vi "Start Trial Assert.vi"(8 "error in":errorcluster, 11 "FPGA VI Ref":T1) -> (0 "error out":errorcluster, 3 "FPGA VI Reference Out":T1)   [LabVIEW 2020]
uses:
  RIG-SPECIFIC FILES/FPGA Refs/FPGA Ref.ctl
  <vilib>/Utility/error.llb/Error Cluster From Error Code.vi
  <vilib>/rvi/errors/niLvFpgaAdjustHostInterfaceError.vi
  <vilib>/rvi/interface/nirviReadWriteControl/nirviReadWriteControl.xnode
  <vilib>/rvi/interface/Simulation/niFpgaSimulationCallBeginRW.vi
  NiFpgaLv.dll
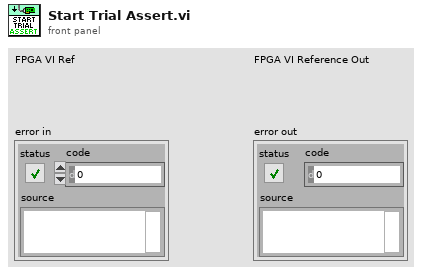
[diagram p1: front panel]
types:
  T1 = typedef "FPGA Ref.ctl" = refnum<k20>
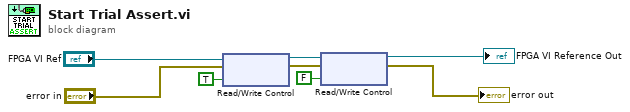
[diagram p0: block diagram]
diagram:
  n1 = xnode "Read/Write Control"("FPGA VI Reference In"="FPGA VI Ref", "error in"="error in", "start_trial"=TRUE) -> ("FPGA VI Reference Out"=w6:T1, "error out"=w5:errorcluster)
  n2 = xnode "Read/Write Control"("FPGA VI Reference In"=w6, "error in"=w5, "start_trial"=FALSE) -> ("FPGA VI Reference Out"=→"FPGA VI Reference Out":T1, "error out"=→"error out":errorcluster)
